vi "DSF.Shared.Configuration.Transfer.Get Channel Configurations.vi"(11 "Transfer Configuration in":refnum<class "DSF.Shared.Configuration.Transfer.lvclass">) -> (2 "Channel Configurations":refnum<class "DSF.Shared.Configuration.Channel.lvclass">[](array[class]), 3 "Transfer Configuration out":refnum<class "DSF.Shared.Configuration.Transfer.lvclass">)   [LabVIEW 2016, in "DSF.Shared.lvlib" / "DSF.Shared.Configuration.Transfer.lvclass"]
uses:
  DSF.Shared.Configuration.Transfer.lvclass
  Channel/DSF.Shared.Configuration.Channel.lvclass
  DSF.Shared.Configuration.Transfer.lvclass/DSF.Shared.Configuration.Transfer.ctl
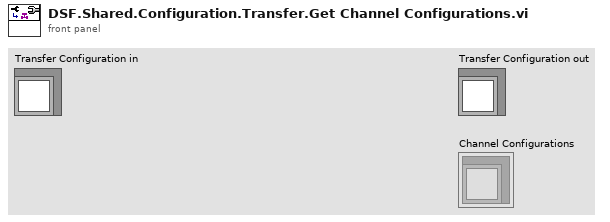
[diagram p1: front panel]
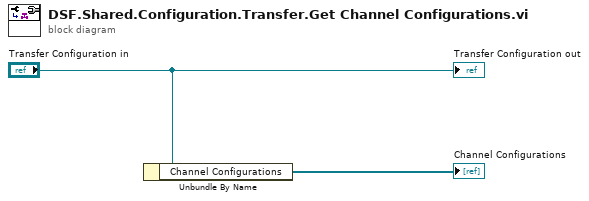
[diagram p0: block diagram]
diagram:
  n1 = Unbundle By Name("Transfer Configuration in") -> ("Channel Configurations"=→"Channel Configurations":refnum<class "DSF.Shared.Configuration.Channel.lvclass">[])
  "Transfer Configuration out" <- "Transfer Configuration in"
